vi "Analysis.Main.vi"(8 "error in (no error)":errorcluster, 10 "Data Path":path, 11 "Parameters":T1={"Results Path"=path "C:/Conti/Logs", "Temp Path"=path "C:/Conti/Temp", "Remote Path"=path "d:/Conti/Logs", "Analysis VIs"=[], "Report Passed?"=FALSE, "Group Channels?"=FALSE}) -> (0 "error out":errorcluster, 3 "Overall Result":bool)   [LabVIEW 2015, in "Analysis.lvlib"]
uses:
  Analysis.lvlib
  Types/Analysis.GUI.Parameters.ctl
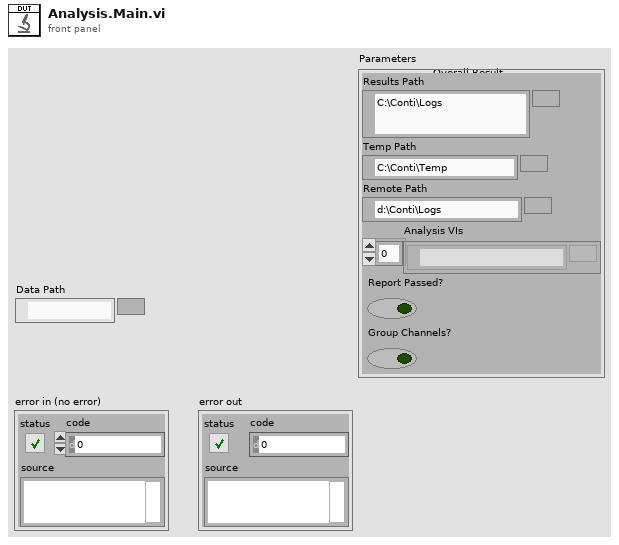
[diagram p1: front panel]
types:
  T1 = typedef "Analysis.lvlib/Analysis.GUI.Parameters.ctl" = cluster{"Results Path":path, "Temp Path":path, "Remote Path":path, "Analysis VIs":path[], "Report Passed?":bool, "Group Channels?":bool}
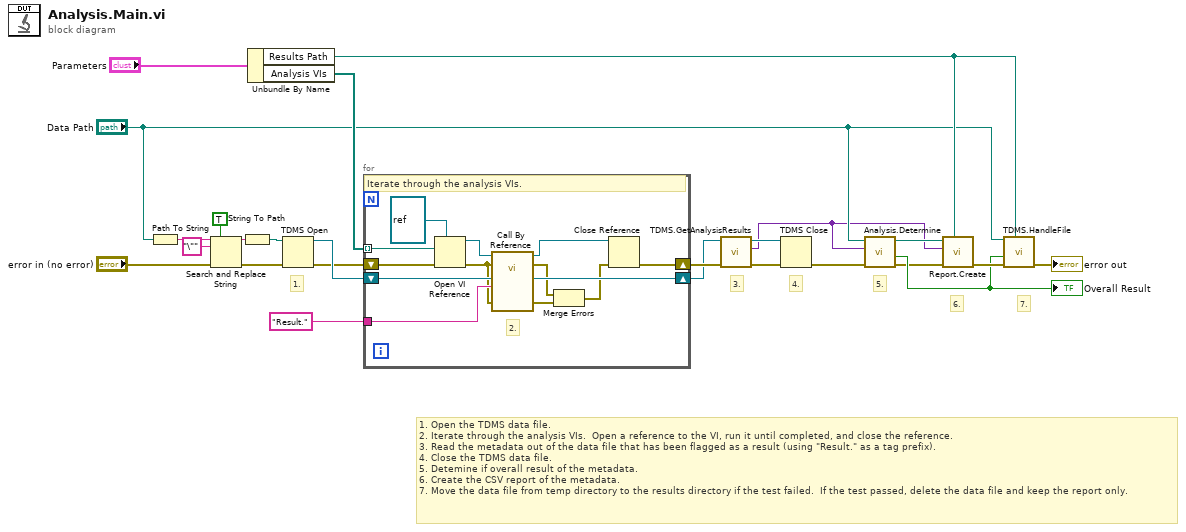
[diagram p0: block diagram]
diagram:
  # "1. Open the TDMS data file.\n2. Iterate through the analysis VIs.  Open a reference to the VI, run it until completed, and close the reference.\n3. Read the metadata out of the data file that has been flagged as a result (using \"Result.\" as a tag prefix).\n4. Close the TDMS data file.\n5. Detemine if overall result of the metadata. \n6. Create the CSV report of the metadata.\n7. Move the data file from temp directory to the results directory if the test failed.  If the test passed, delete the data file and keep the report only."
  # "7."
  # "6."
  # "5."
  # "4."
  # "3."
  # "1."
  n1 = Path To String(path="Data Path") -> (string=w10:string)
  n2 = Search and Replace String(replace all?=TRUE ("replace all? (F)"), input string=w10, search string="\"", error in="error in (no error)") -> (result string=w11:string, error out=w6:errorcluster)  [unwired: 4 in, 2 out]
  n3 = String To Path(string=w11) -> (path=w7:path)
  n4 = Unbundle By Name("Parameters") -> ("Results Path"=w13:path, "Analysis VIs"=w16:path[])
  n5 = TDMS Open(8:w6, 11:w7) -> (0:w2:errorcluster, 3:w3:refnum<k34>)  [unwired: 5 in]
  n6 = for {
    tunnel: "Result." ("Result.Prefix") -> [w36]
    shift-right: [w33] -> w19
    shift-left: w2 -> [w35]
    shift-right: [w31] -> w18
    shift-left: w3 -> [w32]
    tunnel: w16 -> [w26] mode=indexing
    # "2."
    # "Iterate through the analysis VIs."
    n7 = Open VI Reference(type specifier VI Refnum (for type only)=refnum<vi> refnum, vi path=w26, error in (no error)=w35) -> (vi reference=w38:refnum<vi>, error out=w30:errorcluster)  [unwired: 3 in]
    n8 = call-by-ref "?"(reference=w38, error in=w30, "error in"=w30, "Result.Prefix"=w36, "tdms file"=w32) -> (reference out=w34:refnum<vi>, error out=w28:errorcluster, 0:"error out"=w29:errorcluster, "tdms file out"=w31:refnum<k34>)  [unwired: 7 in]
    n9 = Merge Errors(w28, w29) -> (w27:errorcluster)
    n10 = Close Reference(reference=w34, error in (no error)=w27) -> (error out=w33:errorcluster)
  }
  n11 = call "TDMS.GetAnalysisResults.vi"("error in (no error)"=w19, "Refnum in"=w18) -> ("error out"=w23:errorcluster, "Variant"=w1:variant, "Refnum out"=w22:refnum<k34>)  [unwired: 7 in]
  n12 = TDMS Close(8:w23, 11:w22) -> (0:w21:errorcluster)  [unwired: 1 out]
  n13 = call "Analysis.Determine.vi"("error in (no error)"=w21, "Results"=w1, "Data Path"="Data Path") -> ("error out"=w15:errorcluster, "Passed?"=w20:bool, "Data Path"=w14:path)  [unwired: 6 in]
  "Overall Result" <- w20
  n14 = call "Report.Create.vi"("Result Directory"=w13, "error in (no error)"=w15, "Results"=w1, "Data Path"=w14) -> ("error out"=w25:errorcluster)  [unwired: 7 in]
  n15 = call "TDMS.HandleFile.vi"("Result Directory"=w13, "error out"=w25, "Delete"=w20, "Data"="Data Path") -> ("error out"=→"error out":errorcluster)  [unwired: 6 in, 1 out]
